vi "Get Desired Size.vi"(8 "error in (no error)":errorcluster, 11 "Item Summary in":refnum<class "Item Summary.lvclass">) -> (0 "error out":errorcluster, 2 "Desired Size":T1, 3 "Item Summary out":refnum<class "Item Summary.lvclass">)   [LabVIEW 2020, in "Item Summary.lvclass"]
uses:
  Item Summary.lvclass
  <vilib>/IlluminatedG/IG OOPanel/OOPanel/ArrayPanel/Desired Size.ctl
  <vilib>/IlluminatedG/IG OOPanel/OOPanel/OOPanel.lvlib
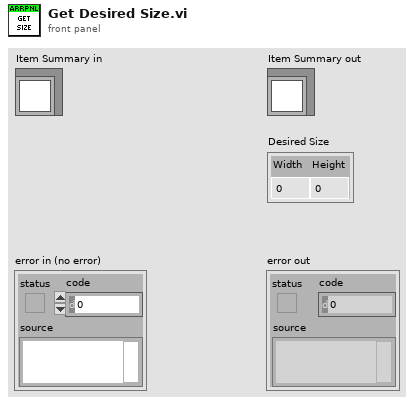
[diagram p1: front panel]
types:
  T1 = typedef "OOPanel.lvlib/Desired Size.ctl" = cluster{"Width":u32, "Height":u32}
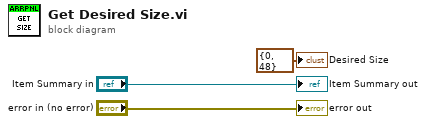
[diagram p0: block diagram]
diagram:
  "error out" <- "error in (no error)"
  "Item Summary out" <- "Item Summary in"
  "Desired Size" <- T1 {"Width"=0, "Height"=48} ("Desired Size")
